vi "Stop Experiment.vi"(8 "error in (no error)":errorcluster, 11 "ExperimentService in":refnum<class "ExperimentService.lvclass">) -> (0 "error out":errorcluster, 3 "ExperimentService out":refnum<class "ExperimentService.lvclass">)   [LabVIEW 2014, in "ExperimentService.lvclass"]
uses:
  ExperimentService.lvclass
  ExperimentService.lvclass/ExperimentService.ctl
  <vilib>/ActorFramework/Message Enqueuer/Message Enqueuer.lvclass/Message Enqueuer.ctl
  <vilib>/ActorFramework/Message Enqueuer/Enqueue.vi
  <vilib>/ActorFramework/Message Priority Queue/Priority Enqueue.vi
  StorageService/StorageService Messages/Save All Msg/Save All Msg.lvclass
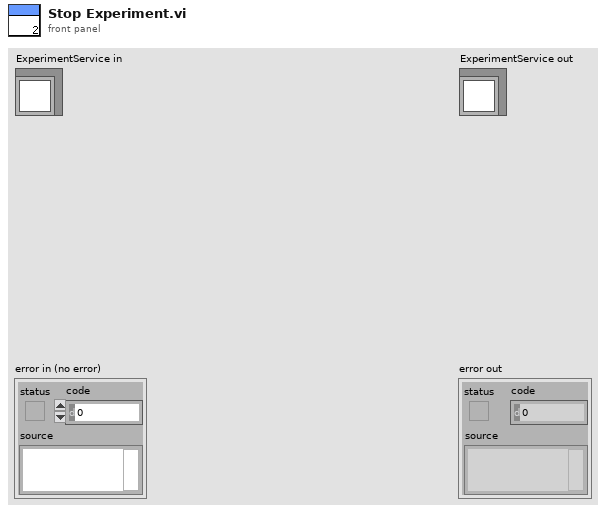
[diagram p1: front panel]
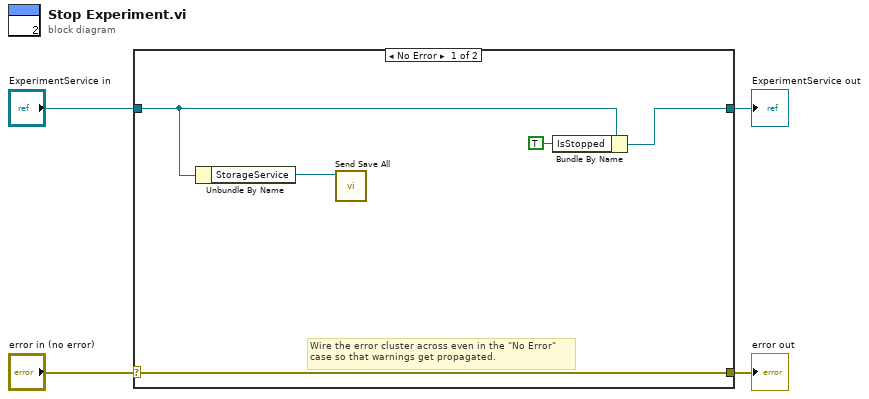
[diagram p0: block diagram]
diagram:
  n1 = case shown="No Error" "error in (no error)" {
    selector: "error in (no error)" -> [w9 w11]
    tunnel: [w9 w11] -> w3
    tunnel: [w6 w10] -> w1
    tunnel: "ExperimentService in" -> [w7 w10]
    frame No Error {
      # "Wire the error cluster across even in the \"No Error\"\ncase so that warnings get propagated."
      n2 = Unbundle By Name(w7) -> ("StorageService"=w8:refnum<class "Message Enqueuer.lvclass">)
      n3 = call "Send Save All.vi"("Message Enqueuer"=w8) -> ()  [unwired: 9 in, 2 out]
      n4 = Bundle By Name(cluster=w7, "IsStopped"=TRUE) -> (w6:refnum<class "ExperimentService.lvclass">)
    }
    frame Error {
    }
  }
  "error out" <- w3
  "ExperimentService out" <- w1
